vi "SPCWriteFile.vi"(5 "Store Path":path, 7 "Data":u16[](array[numeric]), 8 "Error In":errorcluster, 10 "Module No":i16, 11 "DLL Path":path) -> (0 "Error Out":errorcluster, 2 "Module No":i16, 3 "DLL Path":path)   [LabVIEW 2019]
doc: "This function writes the given data to a SPC file. For that it also generates the header for the SPC file. The header are the first four bytes which contains information about the macro time clock and the number of routing channels.\nFor that, the correct module type as well as the correct FIFO type are necessary.\n\nJan 2020\nFrank Quadt\ninfo@becker-hickl.com"
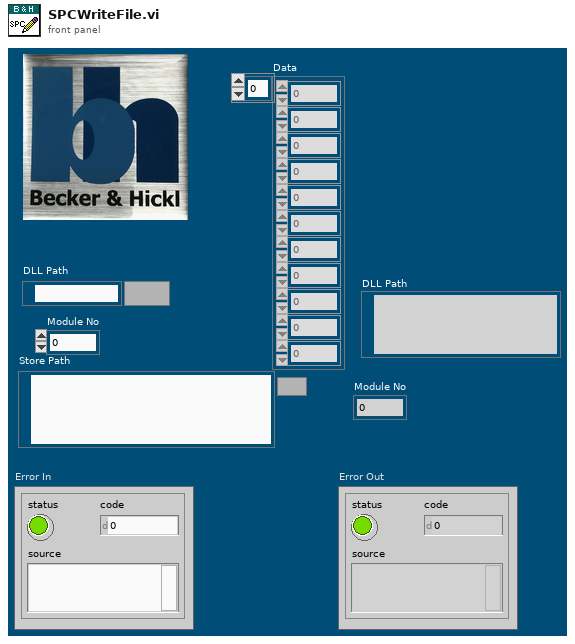
[diagram p1: front panel]
types:
  T1 = enum16{"open", "replace", "create", "open or create", "replace or create", "replace or create with confirmation"}
  T2 = enum16{"big-endian, network order", "native, host order", "little-endian"}
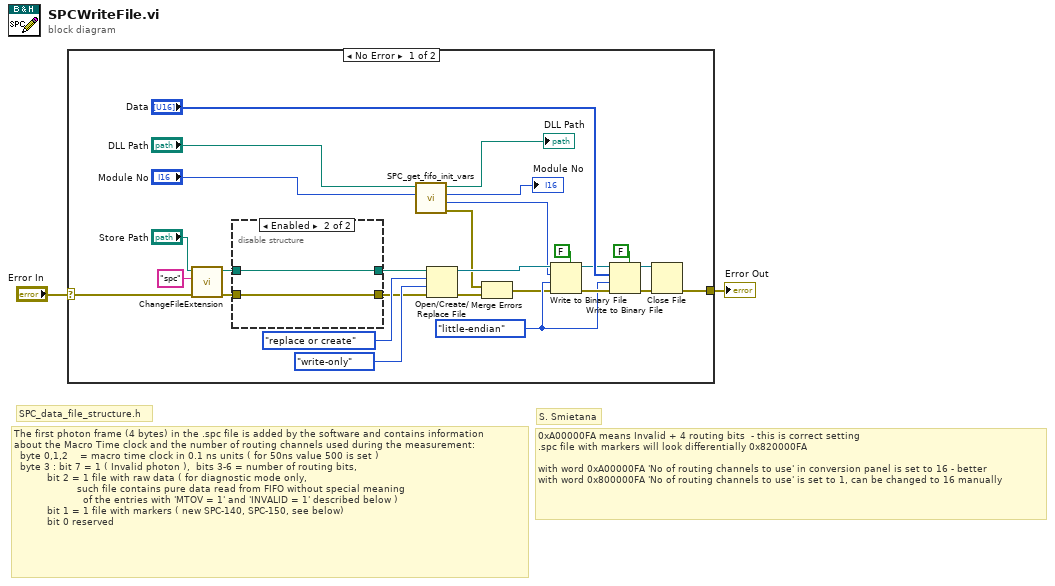
[diagram p0: block diagram]
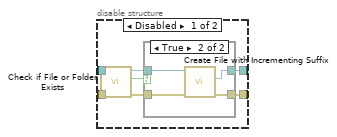
[diagram p2: hidden frame]
diagram:
  # "S. Smietana"
  # "0xA00000FA means Invalid + 4 routing bits  - this is correct setting\n.spc file with markers will look differentially 0x820000FA\n\nwith word 0xA00000FA 'No of routing channels to use' in conversion panel is set to 16 - better\nwith word 0x800000FA 'No of routing channels to use' is set to 1, can be changed to 16 manually"
  # "SPC_data_file_structure.h"
  # "The first photon frame (4 bytes) in the .spc file is added by the software and contains information \nabout the Macro Time clock and the number of routing channels used during the measurement:\n  byte 0,1,2    = macro time clock in 0.1 ns units ( for 50ns value 500 is set )\n  byte 3 : bit 7 = 1 ( Invalid photon ),  bits 3-6 = number of routing bits, \n           bit 2 = 1 file with raw data ( for diagnostic mode only, \n                     such file contains pure data read from FIFO without special meaning \n                       of the entries with 'MTOV = 1' and 'INVALID = 1' described below )\n           bit 1 = 1 file with markers ( new SPC-140, SPC-150, see below)\n           bit 0 reserved"
  n1 = case shown="No Error" "Error In" {
    selector: "Error In" -> [w11 w45]
    tunnel: [w15 w45] -> w2
    frame No Error {
      w18 = T2."little-endian" ("byte order (0:big-endian, network order)")
      n2 = call "ChangeFileExtension.vi"("ErrorIn"=w11, "NewExtension"="spc", "OldPath"="Store Path") -> ("ErrorOut"=w10:errorcluster, "NewPath"=w12:path)  [unwired: 7 in]
      n3 = disable-structure shown="Enabled" {
        disable-tunnel: [w34 w44] -> w23
        disable-tunnel: [w32 w43] -> w22
        disable-tunnel: w12 -> [w31 w44]
        disable-tunnel: w10 -> [w30 w43]
        frame Disabled {
          n4 = call <vilib>:"Check if File or Folder Exists.vi"("error in (no error)"=w30, "path"=w31) -> ("error out"=w33:errorcluster, "file or folder exists?"=w36:bool, "dup path"=w35:path)  [unwired: 7 in]
          n5 = case shown="True" w36 {
            tunnel: w35 -> [w38 w42]
            tunnel: [w38 w41] -> w34
            tunnel: w33 -> [w37 w40]
            tunnel: [w37 w39] -> w32
            frame False {
            }
            frame True {
              n6 = call <vilib>:"Create File with Incrementing Suffix.vi"("error in (no error)"=w40, "file path"=w42) -> ("error out"=w39:errorcluster, "actual path"=w41:path)  [unwired: 7 in, 1 out]
            }
          }
        }
        frame Enabled {
        }
      }
      n7 = call "SPC_get_fifo_init_vars.vi"("Module No."="Module No", "DLL Path"="DLL Path") -> ("Error Out"=w3:errorcluster, "spc_header"=w6:u32, "Module No."=→"Module No":i16, "DLL Path"=→"DLL Path":path)  [unwired: 3 in, 3 out]
      n8 = Open/Create/Replace File(file path (use dialog)=w23, error in=w22, operation (0:open)=T1."replace or create", access (0:read/write)=enum16{"read/write", "read-only", "write-only"}."write-only") -> (refnum out=w27:refnum<file>, error out=w16:errorcluster)  [unwired: 2 in, 1 out]
      n9 = Merge Errors(w3, w16) -> (w14:errorcluster)
      n10 = Write to Binary File(file (use dialog)=w27, data=w6, error in=w14, 5:FALSE, 9:w18) -> (refnum out=w20:refnum<file>, error out=w19:errorcluster)  [unwired: 1 in, 1 out]
      n11 = Write to Binary File(file (use dialog)=w20, data="Data", error in=w19, 5:FALSE ("prepend array or string size? (T)"), 9:w18) -> (refnum out=w28:refnum<file>, error out=w29:errorcluster)  [unwired: 1 in, 1 out]
      n12 = Close File(refnum=w28, error in=w29) -> (error out=w15:errorcluster)  [unwired: 1 out]
    }
    frame Error {
    }
  }
  "Error Out" <- w2
